vi "1WIRE_RESET.vi"(8 "error in":errorcluster) -> (0 "error out":errorcluster, 1 "0 = Device Present / 1=no":bool)   [LabVIEW 2013]
doc: "This VI is created by Vincent Claes for FPDA-1 more information on http://pwo.fpga.be\n\nvincent.claes@xios.be\nclaesvincent@gmail.com\n\nhttp://www.linkedin.com/in/vincentclaes"
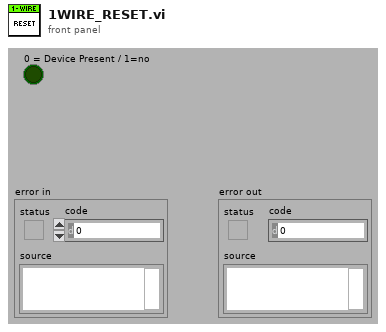
[diagram p1: front panel]
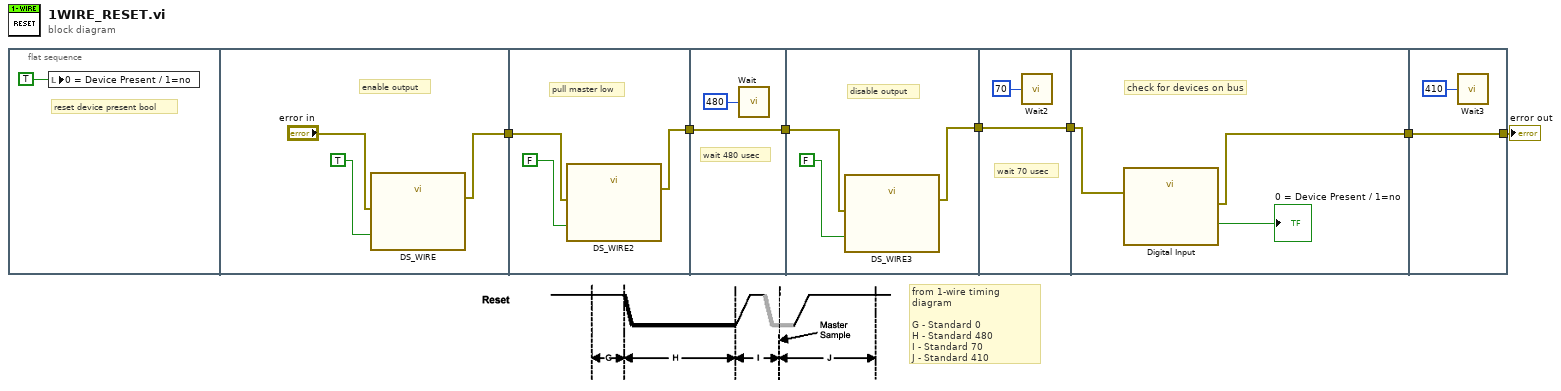
[diagram p0: block diagram]
diagram:
  # "from 1-wire timing diagram\n\nG - Standard 0\nH - Standard 480\nI - Standard 70\nJ - Standard 410"
  n1 = flat-sequence {
    tunnel: [w9] -> w7
    tunnel: w7 -> [w13]
    tunnel: [w12] -> w4
    tunnel: w4 -> [w15]
    tunnel: [w15] -> w3
    tunnel: w3 -> [w18]
    tunnel: [w17] -> w1
    tunnel: [w20] -> w2
    tunnel: w1 -> [w20]
    tunnel: [w22] -> w6
    tunnel: w2 -> [w23]
    tunnel: w6 -> [w25]
    tunnel: [w25] -> w5
    frame #0 {
      # "reset device present bool"
      n2 = local write "0 = Device Present / 1=no"(TRUE ("0 = Device Present / 1=no")) -> ()
    }
    frame #1 {
      # "enable output"
      n3 = call "DS_WIRE"("C/DIO7"=TRUE ("Data"), "error in (no error)"="error in") -> ("error out"=w9:errorcluster)  [unwired: 25 in]
    }
    frame #2 {
      # "pull master low"
      n4 = call "DS_WIRE2"("C/DIO7"=FALSE ("FX2_IO1_J1_0"), "error in (no error)"=w13) -> ("error out"=w12:errorcluster)  [unwired: 25 in]
    }
    frame #3 {
      # "wait 480 usec"
      n5 = call "Wait"("Count(uSec)"=u32 480) -> ()  [unwired: 1 out]
    }
    frame #4 {
      # "disable output"
      n6 = call "DS_WIRE3"("C/DIO7"=FALSE ("Data"), "error in (no error)"=w18) -> ("error out"=w17:errorcluster)  [unwired: 25 in]
    }
    frame #5 {
      # "wait 70 usec"
      n7 = call "Wait2"("Count(uSec)"=u32 70) -> ()  [unwired: 1 out]
    }
    frame #6 {
      # "check for devices on bus"
      n8 = call "Digital Input"("error in (no error)"=w23) -> ("C/DIO7"=→"0 = Device Present / 1=no":bool, "error out"=w22:errorcluster)  [unwired: 25 in]
    }
    frame #7 {
      n9 = call "Wait3"("Count(uSec)"=u32 410) -> ()  [unwired: 1 out]
    }
  }
  "error out" <- w5
